vi "SEN_Loop.vi"() -> ()   [LabVIEW 2020, in "PhotonVision_SEN.lvlib"]
uses:
  PhotonVision_SEN.lvlib
  Utility/Global_STOP.vi
  ENUM_SEN_Action.ctl
  ENUM_SEN_State.ctl
  Global_SEN_Data Out.vi
panel:
  out "Input Bool Data":bool
  out "Output DBL Data":dbl
  out "Cycle Time (S)":dbl format="%.3g"
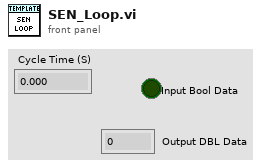
[diagram p1: front panel]
types:
  T1 = typedef "PhotonVision_SEN.lvlib/ENUM_SEN_State.ctl" = enum16{"Startup", "Reset", "Enable", "Disable", "Shutdown"}
  T2 = typedef "PhotonVision_SEN.lvlib/ENUM_SEN_Action.ctl" = enum16{"No Action", "Reset Time", "Reset Enable", "Reset Disable", "Read Enable", "Read Disable"}
  T3 = cluster{"Sensor Ref 0":cluster{i32}, "State":T1, "Previous State":T1, "Current Time":timestamp, "Previous Time":timestamp, "Start Time":timestamp, "Target Time (ms)":u32, "Cycle Time(S)":dbl, "SEN Input":bool, "SEN Output DBL":dbl, "Read Enable":bool}
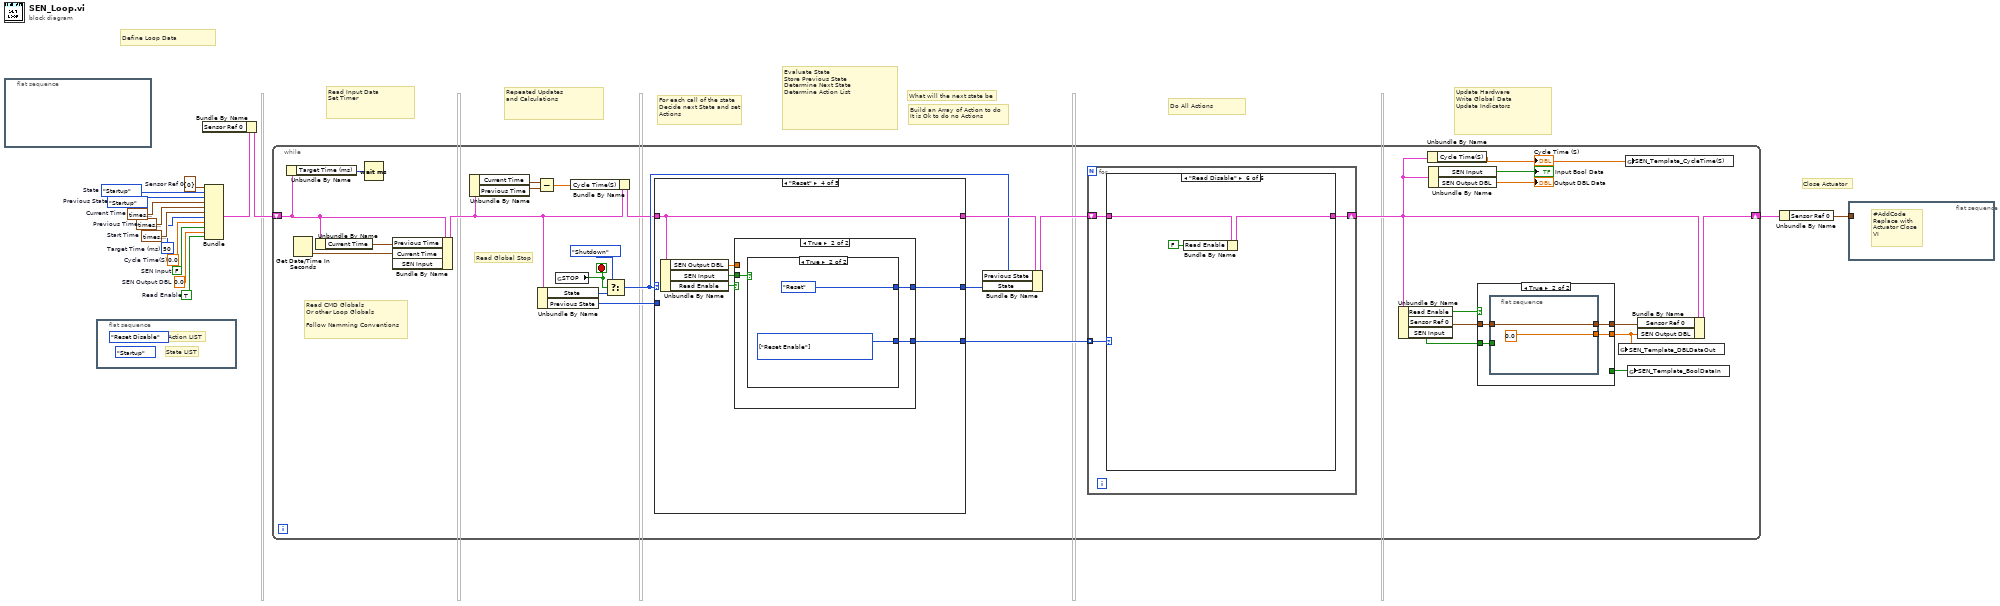
[diagram p0: block diagram]
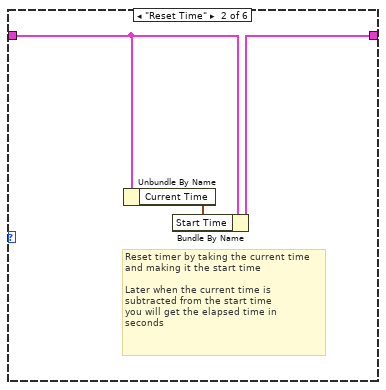
[diagram p4: hidden frame]
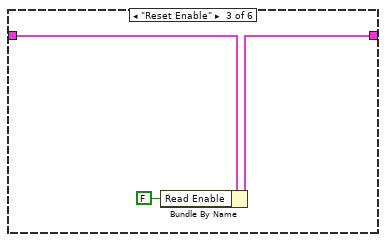
[diagram p5: hidden frame]
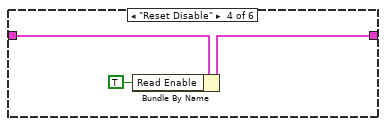
[diagram p6: hidden frame]
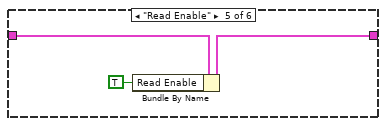
[diagram p7: hidden frame]
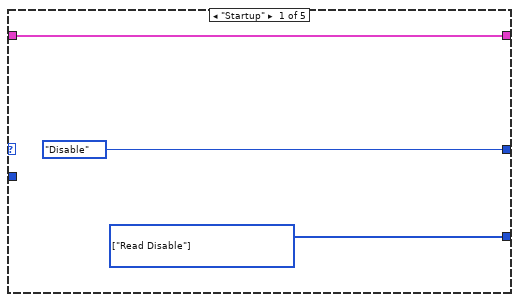
[diagram p8: hidden frame]
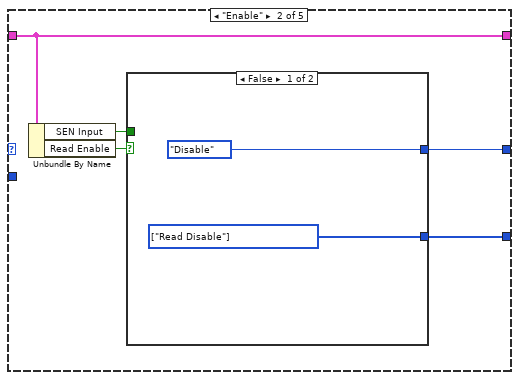
[diagram p9: hidden frame]
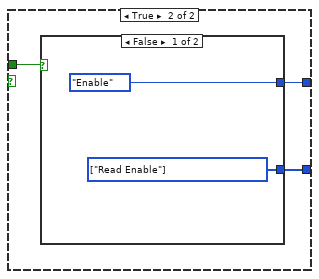
[diagram p10: hidden frame]
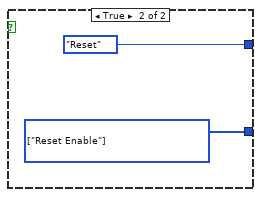
[diagram p11: hidden frame]
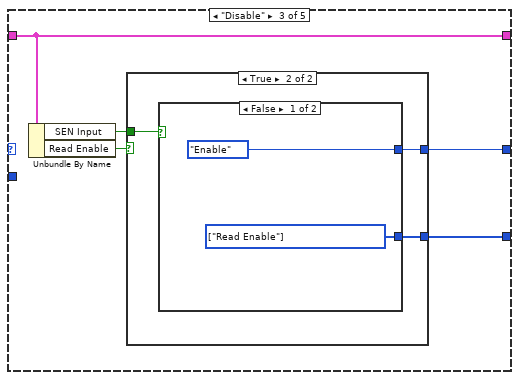
[diagram p12: hidden frame]
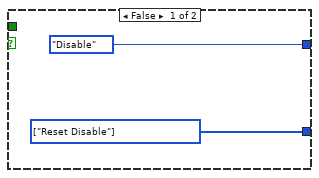
[diagram p13: hidden frame]
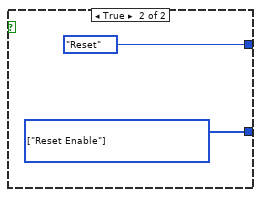
[diagram p14: hidden frame]
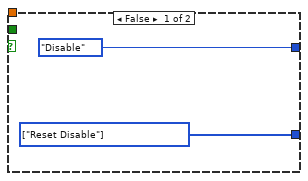
[diagram p15: hidden frame]
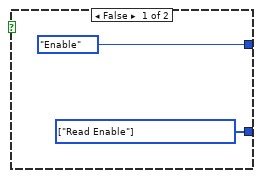
[diagram p16: hidden frame]
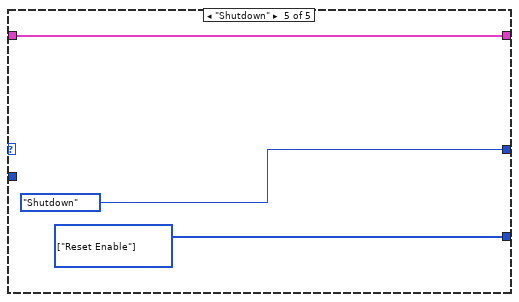
[diagram p17: hidden frame]
diagram:
  w3 = cluster{i32} {0}  # Sensor Ref 0
  w4 = TRUE  # Read Enable
  w7 = 0.0  # Cycle Time(S)
  w8 = ENUM_SEN_State."Startup"  # Previous State
  w9 = timestamp(0 s since 1904-01-01)  # Previous Time
  w10 = u32 50  # Target Time (ms)
  w11 = 0.0  # SEN Output DBL
  w12 = FALSE  # SEN Input
  w13 = timestamp(0 s since 1904-01-01)  # Start Time
  w14 = timestamp(0 s since 1904-01-01)  # Current Time
  w15 = ENUM_SEN_State."Startup"  # State
  # "Build an Array of Action to do\nIt is Ok to do no Actions"
  # "What will the next state be"
  # "For each call of the state\nDecide next State and set\nActions"
  # "Close Actuator"
  # "Define Loop Data"
  # "Repeated Updates\nand Calculations"
  # "Read Input Data\nSet Timer"
  # "Evaluate State\nStore Previous State\nDetermine Next State\nDetermine Action List"
  # "Do All Actions"
  # "Update Hardware\nWrite Global Data\nUpdate Indicators"
  n1 = flat-sequence {
    frame #0 {
    }
  }
  n2 = flat-sequence {
    frame #0 {
      (unwired) ENUM_SEN_State."Startup" ("State")
      (unwired) ENUM_SEN_Action."Reset Disable" ("Action")
      # "State LIST"
      # "Action LIST"
    }
  }
  n3 = Bundle("Sensor Ref 0"=w3, "State"=w15, "Previous State"=w8, "Current Time"=w14, "Previous Time"=w9, "Start Time"=w13, "Target Time (ms)"=w10, "Cycle Time(S)"=w7, "SEN Input"=w12, "SEN Output DBL"=w11, "Read Enable"=w4) -> (w2:T3)  [unwired: 1 in]
  n4 = Bundle By Name(cluster=w2) -> (w1:T3)  [unwired: 1 in]
  n5 = while {
    shift-right: [w21] -> w5
    shift-left: w1 -> [w35]
    stop <- w40 stop-if-true
    # "Read CMD Globals\nOr other Loop Globals\n\nFollow Namming Conventions"
    # "Read Global Stop"
    n6 = Unbundle By Name(w35) -> ("Target Time (ms)"=w37:u32)
    n7 = Get Date/Time In Seconds() -> (seconds since 1Jan1904=w44:timestamp)
    n8 = Unbundle By Name(w35) -> ("Current Time"=w36:timestamp)
    n9 = Wait (ms)(milliseconds to wait=w37) -> ()  [unwired: 1 out]
    n10 = Bundle By Name(cluster=w35, "Previous Time"=w36, "Current Time"=w44) -> (w29:T3)  [unwired: 1 in]
    n11 = Unbundle By Name(w29) -> ("Current Time"=w30:timestamp, "Previous Time"=w31:timestamp)
    n12 = Subtract(x=w30, y=w31) -> (x-y=w27:dbl)
    n13 = Unbundle By Name(w29) -> ("State"=w38:T1, "Previous State"=w34:T1)
    n14 = global read "Global_STOP.vi" "STOP"() -> (w40:bool)
    n15 = Bundle By Name(cluster=w29, "Cycle Time(S)"=w27) -> (w28:T3)
    n16 = Select(t=ENUM_SEN_State."Shutdown" ("State"), s=w40, f=w38) -> (s? t:f=w32:T1)
    n17 = case shown="\"Reset\"" w32 {
      tunnel: w28 -> [w74 w77 w91 w106 w120]
      tunnel: [w74 w77 w91 w106 w120] -> w42
      tunnel: [ENUM_SEN_State."Disable" ("State") w78 w92 w107 ENUM_SEN_State."Shutdown" ("State")] -> w41
      tunnel: [w73 w79 w93 w108 w118] -> w26
      tunnel: w34 -> [_ _ _ _ _]
      frame "Startup" {
        w73 = T2[] [enum."Read Disable"] items=["No Action", "Reset Time", "Reset Enable", "Reset Disable", "Read Enable", "Read Disable"] ("Actions")
      }
      frame "Enable" {
        n18 = Unbundle By Name(w77) -> ("SEN Input"=w75:bool, "Read Enable"=w76:bool)
        n19 = case shown="False" w76 {
          tunnel: [w80 w84] -> w79
          tunnel: [ENUM_SEN_State."Disable" ("State") w83] -> w78
          tunnel: w75 -> [_ w82]
          frame False {
            w80 = T2[] [enum."Read Disable"] items=["No Action", "Reset Time", "Reset Enable", "Reset Disable", "Read Enable", "Read Disable"] ("Actions")
          }
          frame True {
            n20 = case shown="False" w82 {
              tunnel: [w85 w88] -> w84
              tunnel: [ENUM_SEN_State."Enable" ("State") ENUM_SEN_State."Reset" ("State")] -> w83
              frame False {
                w85 = T2[] [enum."Read Enable"] items=["No Action", "Reset Time", "Reset Enable", "Reset Disable", "Read Enable", "Read Disable"] ("Actions")
              }
              frame True {
                w88 = T2[] [enum."Reset Enable"] items=["No Action", "Reset Time", "Reset Enable", "Reset Disable", "Read Enable", "Read Disable"] ("Actions")
              }
            }
          }
        }
      }
      frame "Disable" {
        n21 = Unbundle By Name(w91) -> ("SEN Input"=w89:bool, "Read Enable"=w90:bool)
        n22 = case shown="True" w90 {
          tunnel: [w94 w98] -> w93
          tunnel: [ENUM_SEN_State."Disable" ("State") w97] -> w92
          tunnel: w89 -> [_ w96]
          frame False {
            w94 = T2[] [enum."Reset Disable"] items=["No Action", "Reset Time", "Reset Enable", "Reset Disable", "Read Enable", "Read Disable"] ("Actions")
          }
          frame True {
            n23 = case shown="False" w96 {
              tunnel: [w99 w102] -> w98
              tunnel: [ENUM_SEN_State."Enable" ("State") ENUM_SEN_State."Reset" ("State")] -> w97
              frame False {
                w99 = T2[] [enum."Read Enable"] items=["No Action", "Reset Time", "Reset Enable", "Reset Disable", "Read Enable", "Read Disable"] ("Actions")
              }
              frame True {
                w102 = T2[] [enum."Reset Enable"] items=["No Action", "Reset Time", "Reset Enable", "Reset Disable", "Read Enable", "Read Disable"] ("Actions")
              }
            }
          }
        }
      }
      frame "Reset" {
        n24 = Unbundle By Name(w106) -> ("SEN Output DBL"=w103:dbl, "SEN Input"=w104:bool, "Read Enable"=w105:bool)
        n25 = case shown="True" w105 {
          tunnel: [w109 w113] -> w108
          tunnel: [ENUM_SEN_State."Disable" ("State") w112] -> w107
          tunnel: w104 -> [_ w111]
          tunnel: w103 -> [_ _]
          frame False {
            w109 = T2[] [enum."Reset Disable"] items=["No Action", "Reset Time", "Reset Enable", "Reset Disable", "Read Enable", "Read Disable"] ("Actions")
          }
          frame True {
            n26 = case shown="True" w111 {
              tunnel: [w114 w117] -> w113
              tunnel: [ENUM_SEN_State."Enable" ("State") ENUM_SEN_State."Reset" ("State")] -> w112
              frame False {
                w114 = T2[] [enum."Read Enable"] items=["No Action", "Reset Time", "Reset Enable", "Reset Disable", "Read Enable", "Read Disable"] ("Actions")
              }
              frame True {
                w117 = T2[] [enum."Reset Enable"] items=["No Action", "Reset Time", "Reset Enable", "Reset Disable", "Read Enable", "Read Disable"] ("Actions")
              }
            }
          }
        }
      }
      frame "Shutdown" {
        w118 = T2[] [enum."Reset Enable"] items=["No Action", "Reset Time", "Reset Enable", "Reset Disable", "Read Enable", "Read Disable"] ("Actions")
      }
    }
    n27 = Bundle By Name(cluster=w42, "Previous State"=w32, "State"=w41) -> (w43:T3)
    n28 = for {
      tunnel: w26 -> [w55] mode=indexing
      shift-right: [w54] -> w22
      shift-left: w43 -> [w53]
      n29 = case shown="\"Read Disable\"" w55 {
        tunnel: w53 -> [w56 w59 w62 w65 w68 w71]
        tunnel: [w56 w58 w61 w64 w67 w70] -> w54
        frame "No Action" {
        }
        frame "Reset Time" {
          # "Reset timer by taking the current time\nand making it the start time\n\nLater when the current time is \nsubtracted from the start time\nyou will get the elapsed time in \nseconds"
          n30 = Unbundle By Name(w59) -> ("Current Time"=w57:timestamp)
          n31 = Bundle By Name(cluster=w59, "Start Time"=w57) -> (w58:T3)
        }
        frame "Reset Enable" {
          n32 = Bundle By Name(cluster=w62, "Read Enable"=FALSE) -> (w61:T3)
        }
        frame "Reset Disable" {
          n33 = Bundle By Name(cluster=w65, "Read Enable"=TRUE) -> (w64:T3)
        }
        frame "Read Enable" {
          n34 = Bundle By Name(cluster=w68, "Read Enable"=TRUE) -> (w67:T3)
        }
        frame "Read Disable" {
          n35 = Bundle By Name(cluster=w71, "Read Enable"=FALSE) -> (w70:T3)
        }
      }
    }
    n36 = Unbundle By Name(w22) -> ("Read Enable"=w18:bool, "Sensor Ref 0"=w24:cluster{i32}, "SEN Input"=w17:bool)
    n37 = Unbundle By Name(w22) -> ("Cycle Time(S)"=w20:dbl)
    "Cycle Time (S)" <- w20
    n38 = Unbundle By Name(w22) -> ("SEN Input"=→"Input Bool Data":bool, "SEN Output DBL"=→"Output DBL Data":dbl)
    n39 = case shown="True" w18 {
      tunnel: w24 -> [w46 w50]
      tunnel: [w46 w49] -> w23
      tunnel: [_ w48] -> w19
      tunnel: w17 -> [w45 w47]
      tunnel: [w45 _] -> w16
      frame False {
      }
      frame True {
        n40 = flat-sequence {
          tunnel: w50 -> [w52]
          tunnel: [w52] -> w49
          tunnel: [0.0 ("ACT_Template_DBLDataOut")] -> w48
          tunnel: w47 -> [_]
          frame #0 {
          }
        }
      }
    }
    n41 = global write "Global_SEN_Data Out.vi" "SEN_Template_DBLDataOut"(w19) -> ()
    n42 = global write "Global_SEN_Data Out.vi" "SEN_Template_CycleTime(S)"(w20) -> ()
    n43 = global write "Global_SEN_Data Out.vi" "SEN_Template_BoolDataIn"(w16) -> ()
    n44 = Bundle By Name(cluster=w22, "Sensor Ref 0"=w23, "SEN Output DBL"=w19) -> (w21:T3)
  }
  n45 = Unbundle By Name(w5) -> ("Sensor Ref 0"=w6:cluster{i32})
  n46 = flat-sequence {
    tunnel: w6 -> [_]
    frame #0 {
      # "#AddCode\nReplace with \nActuator Close\nVI"
    }
  }
